vi "Test-Forget Error.vi"   [LabVIEW 2017]
uses:
  src/Dialog Type.ctl
  <vilib>/addons/_JKI Toolkits/Caraya/classes/Assert/Assert Less_Variant.vi
  <vilib>/addons/_JKI Toolkits/Caraya/classes/Assert/Assert Error.vi
  <vilib>/addons/_JKI Toolkits/Caraya/classes/Test/Test.lvclass
  <vilib>/addons/_JKI Toolkits/Caraya/classes/Assert/Assert.lvclass
  src/Error Dialog w Copy to Clipboard.lvlib
types:
  T1 = typedef "Error Dialog w Copy to Clipboard.lvlib/Dialog Type.ctl" = enum16{"OK message", "Continue or Stop message"}
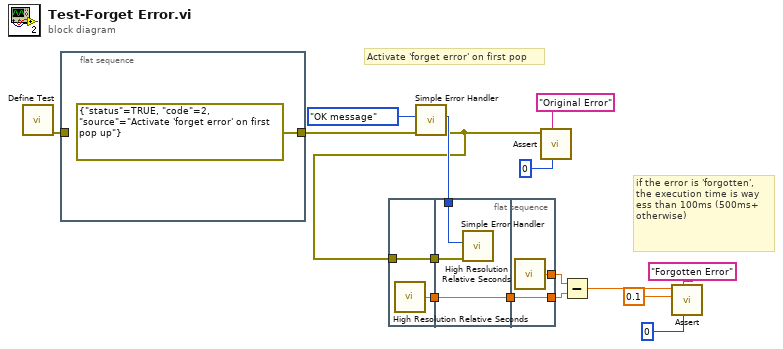
[diagram p0: block diagram]
diagram:
  w11 = Dialog_Type."OK message" ("Dialog Type")
  # "if the error is 'forgotten',\nthe execution time is way \ness than 100ms (500ms+\notherwise)"
  # "Activate 'forget error' on first pop"
  n1 = call <vilib>:"Define Test.vi"() -> ("error out"=w10:errorcluster)  [unwired: 11 in]
  n2 = flat-sequence {
    tunnel: w10 -> [_]
    tunnel: [errorcluster {"status"=TRUE, "code"=2, "source"="Activate 'forget error' on first pop up"} ("error out")] -> w9
    frame #0 {
    }
  }
  n3 = flat-sequence {
    tunnel: w8 -> [w18]
    tunnel: [w18] -> w7
    tunnel: [w17] -> w5
    tunnel: w11 -> [w21]
    tunnel: w7 -> [w20]
    tunnel: [w19] -> w6
    tunnel: w5 -> [w19]
    tunnel: [w23] -> w4
    tunnel: [w22] -> w3
    tunnel: w6 -> [w22]
    frame #0 {
      n4 = call <vilib>:"High Resolution Relative Seconds.vi"() -> ("relative seconds"=w17:dbl)
    }
    frame #1 {
      n5 = call "Simple Error Handler.vi"("error in (no error)"=w20, "Dialog Type"=w21) -> ()  [unwired: 9 in, 1 out]
    }
    frame #2 {
      n6 = call <vilib>:"High Resolution Relative Seconds.vi"() -> ("relative seconds"=w23:dbl)
    }
  }
  n7 = call "Simple Error Handler.vi"("error in (no error)"=w9, "Dialog Type"=w11) -> ("error out"=w8:errorcluster)  [unwired: 9 in]
  n8 = call-poly <vilib>:"Assert.vi"("error code (1)"=0, "Label"="Original Error", "Error?"=w8) -> ()  [unwired: 8 in, 1 out]
  n9 = Subtract(x=w4, y=w3) -> (x-y=w2:dbl)
  n10 = call-poly <vilib>:"Assert.vi"("error code (1)"=0, "Label"="Forgotten Error", "Y"=0.1 ("x-y"), "X"=w2) -> ()  [unwired: 7 in, 1 out]
